vi "update status string.vi"(8 "error in":errorcluster, 11 "Consumer Cluster in":T1={"This VI Ref"=refnum, "Test VI"=refnum, "Q Ref"=refnum, "UE"=refnum, "Data"=variant, "Timeout"=-1, "Path List[]"=[], "Status"="", "Counter"=0, "Config"={"Source Path"=path "", "Dest Path"=path "", "Log Path"=path "", "Move?"=FALSE, "Log?"=FALSE, "Scanners"=[], "Excude Folders"=[], "Jpg?"=FALSE, "Default path"=path "", "Extended?"=FALSE, "Mode"=enum."Move"}, "Total"=0, "Config Path"=path "", "exif info"={"Make"="Canon\u0000", "Model"="Canon PowerShot A495\u0000", "Orientation"=0, "Date"=timestamp(0 s since 1904-01-01), "Width"=0, "Height"=0, "Square?"=FALSE, "File Name"="Canon\u0000", "Extension"="Canon\u0000", "Valid?"=FALSE, "Path"=path "", "size"=0, "No Ext?"=FALSE, "prefix?"=FALSE, "String"="", "Name Type"=enum."Event Sufix"}, "app operation"=enum."Start", "Log Ref"=refnum, "Start Time"=0.0, "Pause Time"=0.0, "Argument?"=FALSE, "Argument path"=path "", "Identical"=FALSE, "File.lvclass"=refnum}) -> (0 "error out":errorcluster, 1 "String":string, 3 "cluster out":T1={"This VI Ref"=refnum, "Test VI"=refnum, "Q Ref"=refnum, "UE"=refnum, "Data"=variant, "Timeout"=-1, "Path List[]"=[], "Status"="", "Counter"=0, "Config"={"Source Path"=path "", "Dest Path"=path "", "Log Path"=path "", "Move?"=FALSE, "Log?"=FALSE, "Scanners"=[], "Excude Folders"=[], "Jpg?"=FALSE, "Default path"=path "", "Extended?"=FALSE, "Mode"=enum."Move"}, "Total"=0, "Config Path"=path "", "exif info"={"Make"="Canon\u0000", "Model"="Canon PowerShot A495\u0000", "Orientation"=0, "Date"=timestamp(0 s since 1904-01-01), "Width"=0, "Height"=0, "Square?"=FALSE, "File Name"="Canon\u0000", "Extension"="Canon\u0000", "Valid?"=FALSE, "Path"=path "", "size"=0, "No Ext?"=FALSE, "prefix?"=FALSE, "String"="", "Name Type"=enum."Event Sufix"}, "app operation"=enum."Start", "Log Ref"=refnum, "Start Time"=0.0, "Pause Time"=0.0, "Argument?"=FALSE, "Argument path"=path "", "Identical"=FALSE, "File.lvclass"=refnum}, 4 "Slide":dbl(slide) scale=0.0..100.0)   [LabVIEW 2023, in "User Interface.lvlib"]
uses:
  User Interface.lvlib
  Controls/main consumer cluster.ctl
  File Classes/File/File.lvclass
  Controls/configuration cluster.ctl
  File Classes/Controls/exif data cluster.ctl
  File Classes/Controls/rename type enum.ctl
  Controls/app operation state enum.ctl
  File Classes/File Classes.lvlib
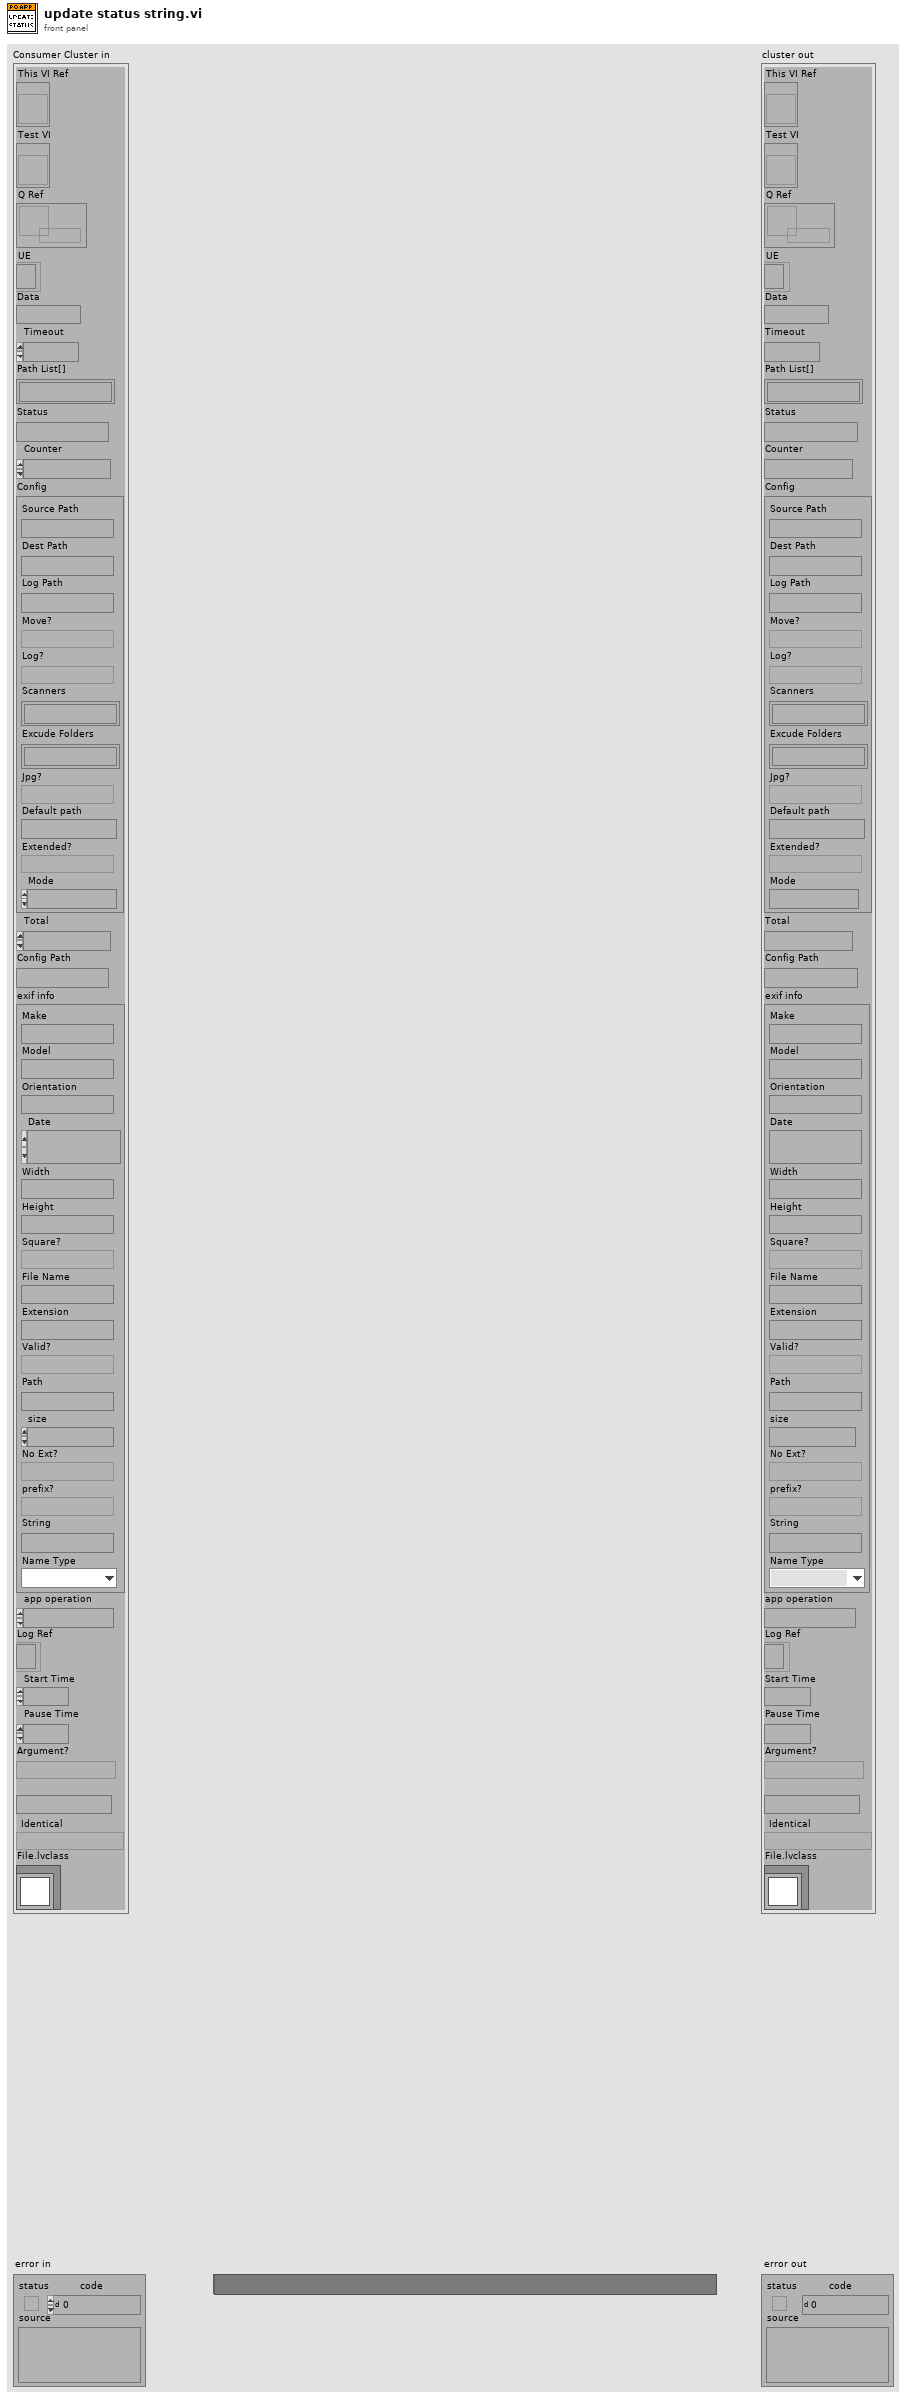
[diagram p1: front panel]
types:
  T1 = typedef "User Interface.lvlib/main consumer cluster.ctl" = cluster{"This VI Ref":refnum<vi>, "Test VI":refnum<vi>, "Q Ref":refnum<queue>, "UE":refnum<event-registration>, "Data":variant, "Timeout":i32, "Path List[]":path[], "Status":string, "Counter":i32, "Config":T2, "Total":i32, "Config Path":path, "exif info":T3, "app operation":T5, "Log Ref":refnum<file>, "Start Time":dbl, "Pause Time":dbl, "Argument?":bool, "Argument path":path, "Identical":bool, "File.lvclass":refnum<class "File.lvclass">}
  T2 = typedef "User Interface.lvlib/configuration cluster.ctl" = cluster{"Source Path":path, "Dest Path":path, "Log Path":path, "Move?":bool, "Log?":bool, "Scanners":string[], "Excude Folders":string[], "Jpg?":bool, "Default path":path, "Extended?":bool, "Mode":enum16{"Copy (Default)", "Move", "Rename"}}
  T3 = typedef "File Classes.lvlib/exif data cluster.ctl" = cluster{"Make":string, "Model":string, "Orientation":u16, "Date":timestamp, "Width":u16, "Height":u16, "Square?":bool, "File Name":string, "Extension":string, "Valid?":bool, "Path":path, "size":i64, "No Ext?":bool, "prefix?":bool, "String":string, "Name Type":T4}
  T4 = typedef "File Classes.lvlib/rename type enum.ctl" = enum16{"Date & Time (Default)", "Model Sufix", "Event Sufix", "Model & Event Sufix"}
  T5 = typedef "User Interface.lvlib/app operation state enum.ctl" = enum16{"Start", "Stop", "Pause", "Resume"}
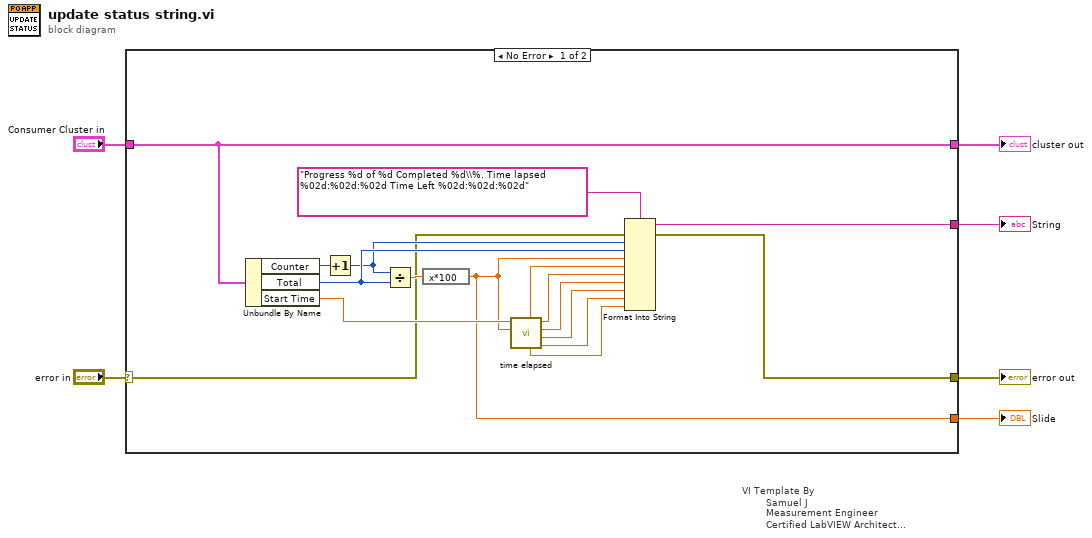
[diagram p0: block diagram]
diagram:
  n1 = case "VI Template By\n        Samuel J\n        Measurement Engineer\n        Certified LabVIEW Architect\n        Vestas Technology R&D Chennai" shown="No Error" "error in" {
    selector: "error in" -> [w10 w25]
    tunnel: [w9 w25] -> w5
    tunnel: [w11 w24] -> w3
    tunnel: "Consumer Cluster in" -> [w11 w24]
    tunnel: [w8 _] -> w2
    tunnel: [w7 _] -> w1
    frame No Error {
      n2 = Unbundle By Name(w11) -> ("Counter"=w21:i32, "Total"=w22:i32, "Start Time"=w18:dbl)
      n3 = Increment(x=w21) -> (x+1=w19:i32)
      n4 = Divide(x=w19, y=w22) -> (x/y=w20:dbl)
      n5 = expression code="x*100"(w20) -> (w7:dbl)
      n6 = call "time elapsed.vi"("%Completed"=w7, "Start"=w18) -> ("Minuites 2"=w13:dbl, "Hours 2"=w14:dbl, "Seconds"=w15:dbl, "Minuites"=w16:dbl, "Seconds 2"=w12:dbl, "Hours"=w17:dbl)  [unwired: 4 in]
      n7 = Format Into String(format string="Progress %d of %d Completed %d\\%. Time lapsed %02d:%02d:%02d Time Left %02d:%02d:%02d", error in=w10, w19, w22, w7, w17, w16, w15, w14, w13, w12) -> (resulting string=w8:string, error out=w9:errorcluster)  [unwired: 1 in]
    }
    frame Error {
    }
  }
  "error out" <- w5
  "cluster out" <- w3
  "String" <- w2
  "Slide" <- w1
